vi "Create Error Enqueuer.vi"(8 "error in (no error)":errorcluster) -> (0 "error out":errorcluster, 2 "Error Enqueuer":refnum<user-event>, 3 "Messages":refnum<event-registration>)   [LabVIEW 2018, in "Actor.lvclass"]
uses:
  Actor.lvclass
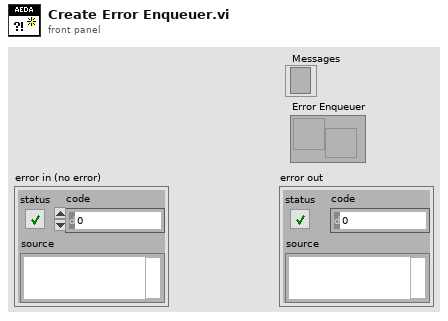
[diagram p1: front panel]
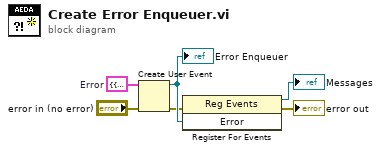
[diagram p0: block diagram]
diagram:
  w3 = cluster{"Error":errorcluster} {"Error"={"status"=FALSE, "code"=0, "source"=""}}  # Error
  n1 = Create User Event(user event datatype=w3, error in="error in (no error)") -> (user event=w5:refnum<user-event>, error out=w4:errorcluster)
  "Error Enqueuer" <- w5
  n2 = register-events(error in=w4, w5) -> (reference out=→"Messages":refnum<event-registration>, error out=→"error out":errorcluster)  [unwired: 1 in]
